vi "Measurement Done.vi"(6 "Array of Hardware":refnum<class "Hardware.lvclass">[](array[class]), 8 "error in (no error)":errorcluster, 9 "Measurement Name":string, 10 "GUID":string, 11 "Client Controller in":refnum<class "Client Controller.lvclass">) -> (0 "error out":errorcluster, 3 "Client Controller out":refnum<class "Client Controller.lvclass">)   [LabVIEW 2017, in "Client Controller.lvlib" / "Client Controller.lvclass"]
uses:
  Client Controller.lvclass
  MAL-Framework/user.lib/Common Components/Hardware/Hardware.lvclass
  MAL-Framework/user.lib/Common Components/Controller/Controller.lvclass
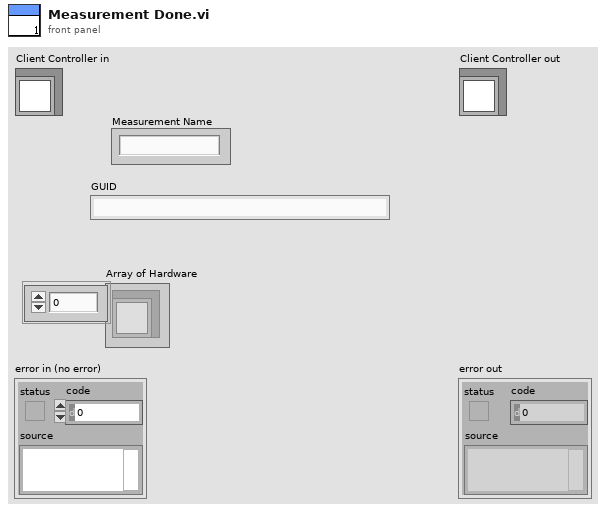
[diagram p1: front panel]
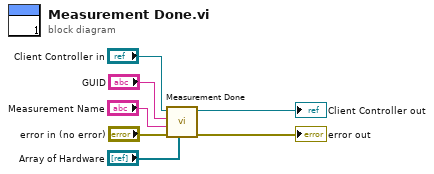
[diagram p0: block diagram]
diagram:
  n1 = call-parent "Measurement Done.vi"("Array of Hardware"="Array of Hardware", "error in (no error)"="error in (no error)", "Measurement Name"="Measurement Name", "GUID"="GUID", "Controller in"="Client Controller in") -> ("error out"=→"error out":errorcluster, "Controller out"=→"Client Controller out":refnum<class "Client Controller.lvclass">)  [unwired: 5 in]
